vi "Main Page.vi"(8 "error in (no error)":errorcluster, 11 "Node Ptr":T2 format="%.0x") -> (0 "error out":errorcluster)   [LabVIEW 2014, in "SLSC configuration System Explorer.lvlib"]
uses:
  SLSC configuration System Explorer.lvlib
  <vilib>/NI Veristand/Custom Device API/Custom Device Item Ref.ctl
  Shared/Type Defs/RIO Device Address.ctl
  Type Defs/Card Position.ctl
  Example/SPI Utility/Slot #.ctl
  <vilib>/NI Veristand/Custom Device API/Dependent File Optional Info.ctl
  Shared/Constants.vi
  <vilib>/NI Veristand/Custom Device API/Get Item Property (U16).vi
  <vilib>/NI Veristand/Custom Device API/Get Item Property (U32).vi
  <vilib>/NI Veristand/Custom Device API/Get Item Property (Dependent File).vi
  <vilib>/NI Veristand/Custom Device API/Get Item Property (String).vi
  <vilib>/NI Veristand/Custom Device API/Set Item Property (U16).vi
  <vilib>/NI Veristand/Custom Device API/Set Item Property (U32).vi
  <vilib>/NI Veristand/Custom Device API/Set Item Property (Dependent File).vi
  <vilib>/NI Veristand/Custom Device API/Set Item Property (String).vi
  <vilib>/NI Veristand/Custom Device API/Custom Device API.lvlib
  Shared/SLSC configuration Shared.lvlib
panel:
  in  "Header 5":cluster{"Section Name":string}={"Section Name"="Slot Configuration"}
  out "Slot Configuration":string[][](table)
  out "SPI Clock Frequency (Hz)":dbl
  in  "Sample Rate (S/s)":u32 min=1 max=40000000
  in  "FPGA Load Delay (s)":u8
  in  "SPI Divide Value":u8 min=1
  in  "Header 4":cluster{"Section Name":string}={"Section Name"="SPI Configuration"}
  in  "Header 3":cluster{"Section Name":string}={"Section Name"="FPGA Configuration"}
  in  "Header 2":cluster{"Section Name":string}={"Section Name"="Device Settings"}
  in  "RIO Device Address":T1="RIO0"
  in  "Path":path
  in  "Header":cluster{"Section Name":string}={"Section Name"="SLSC Custom Device Settings"}
  in  "Name":string
  # "120 MHz"
  # "______________________"
  # "SPI Clock Frequency ="
  # "(Divide Value + 1) x 2"
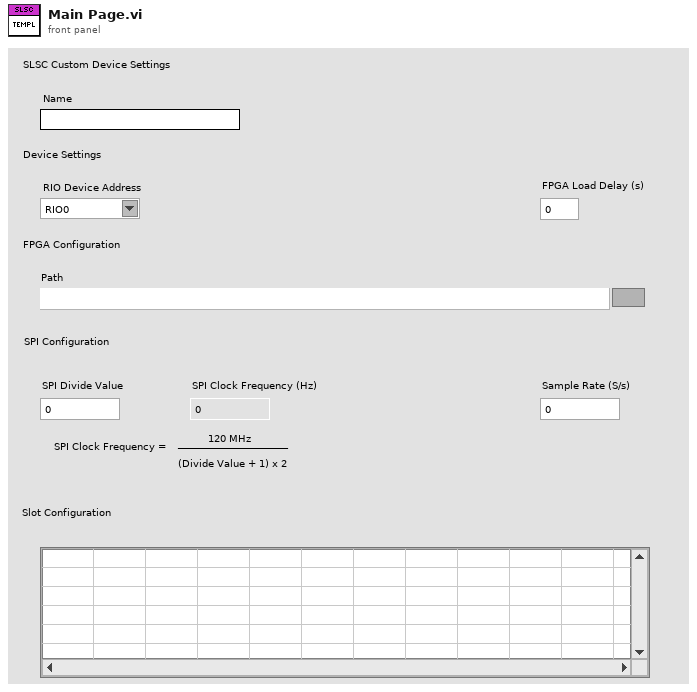
[diagram p1: front panel]
types:
  T1 = typedef "SLSC configuration System Explorer.lvlib/RIO Device Address.ctl" = string
  T2 = typedef "Custom Device API.lvlib/Custom Device Item Ref.ctl" = u64
  T3 = typedef "SLSC configuration Shared.lvlib/Card Position.ctl" = cluster{"Rack #":u8, "Slot #":T4}
  T4 = typedef "SLSC configuration Shared.lvlib/Slot #.ctl" = u8
  T5 = typedef "Custom Device API.lvlib/Custom Device Item Info.ctl" = cluster{"Name":string, "Is Channel":bool, "GUID":string, "Is Waveform":bool}
  T6 = typedef "Custom Device API.lvlib/Dependent File Optional Info.ctl" = cluster{"Version":string, "RTDestination":path, "ForceDownload":bool, "SupportedTarget":string, "MD5":string}
  T7 = typedef "Custom Device API.lvlib/Custom Device Commands.ctl" = enum16{"Default", "Item renamed", "Shutdown", "Dynamic button pressed"}
  T8 = typedef "LVPoint32TypeDef.ctl" = cluster{"Horizontal":i32, "Vertical":i32}
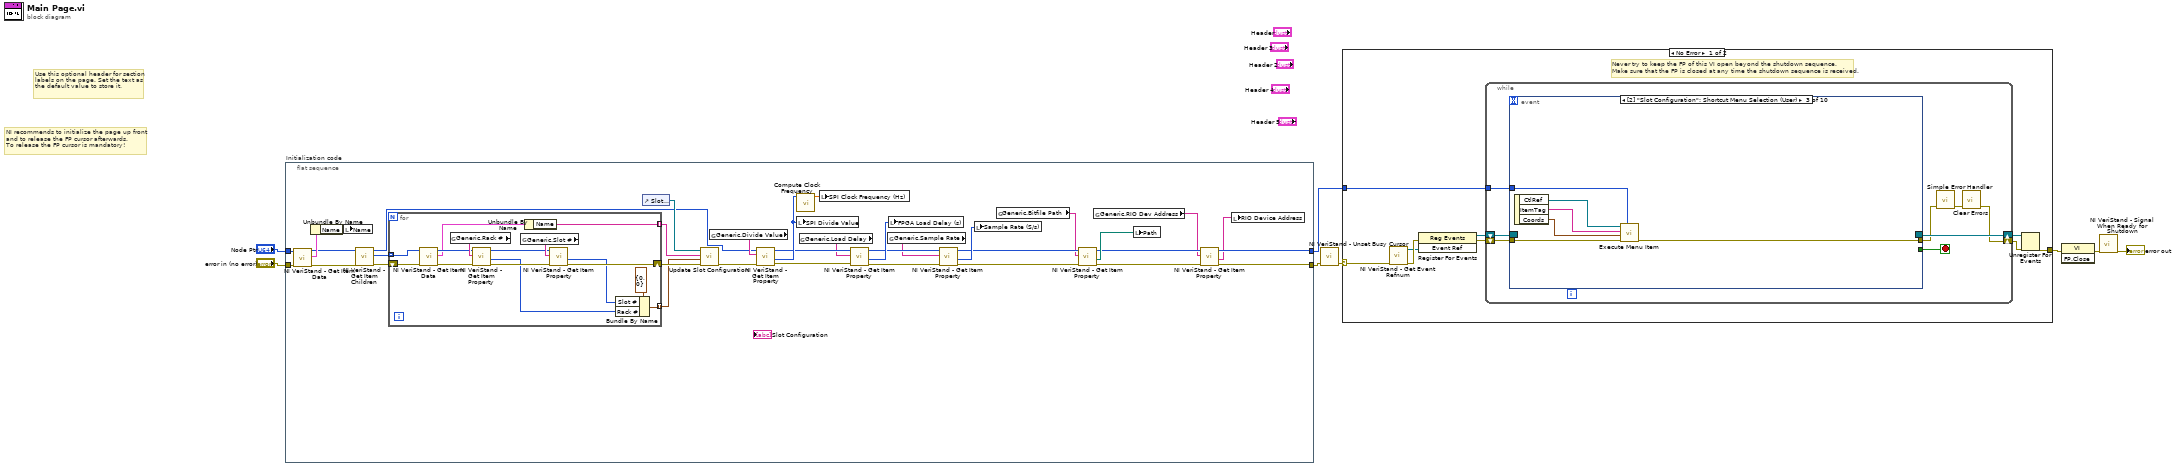
[diagram p0: block diagram]
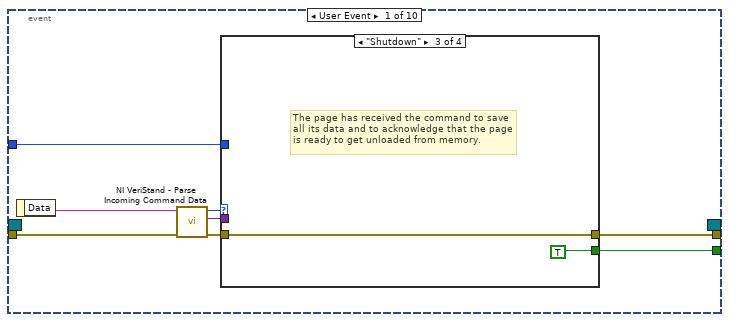
[diagram p2: hidden frame]
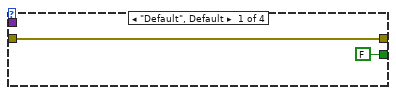
[diagram p3: hidden frame]
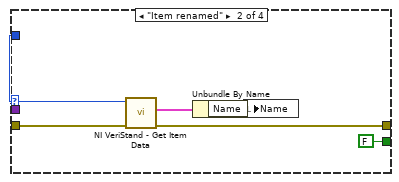
[diagram p4: hidden frame]
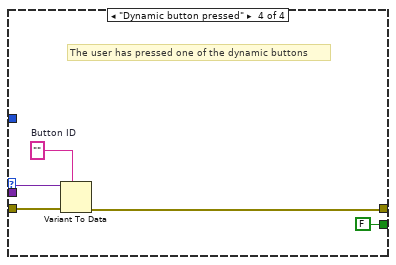
[diagram p5: hidden frame]
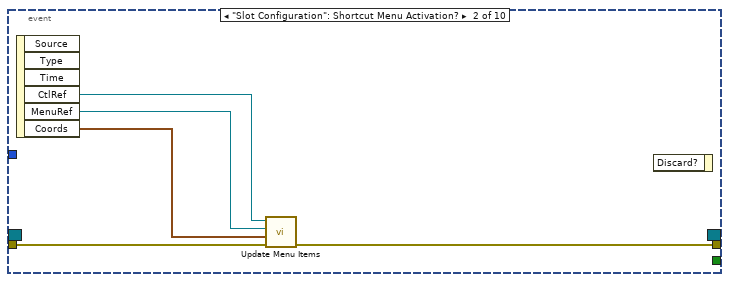
[diagram p6: hidden frame]
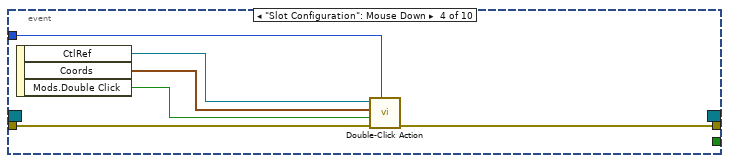
[diagram p7: hidden frame]
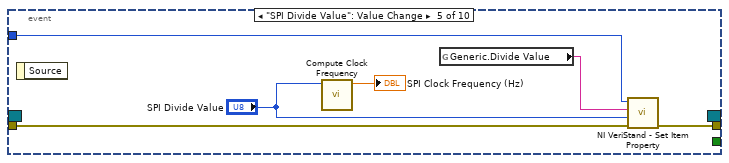
[diagram p8: hidden frame]
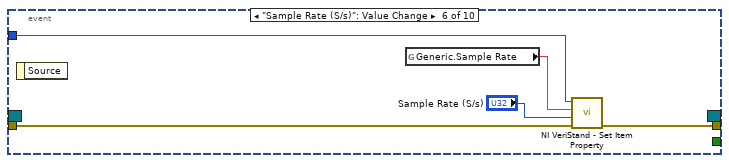
[diagram p9: hidden frame]
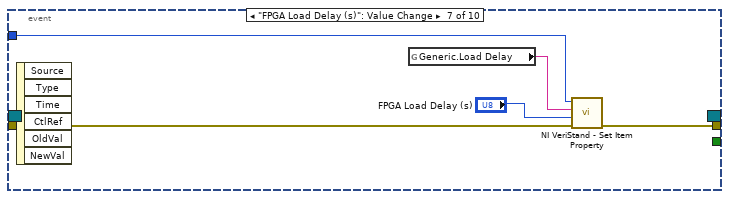
[diagram p10: hidden frame]
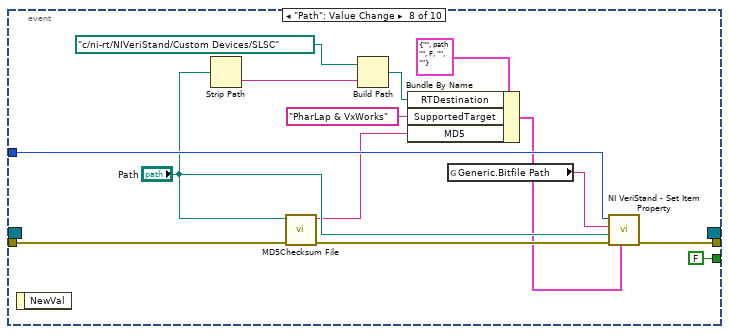
[diagram p11: hidden frame]
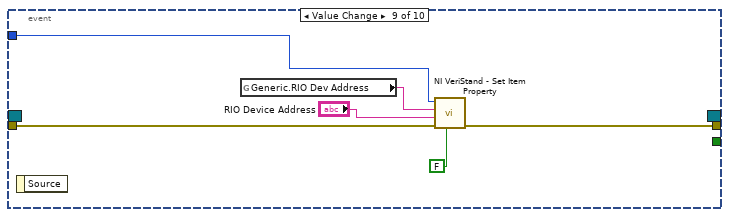
[diagram p12: hidden frame]
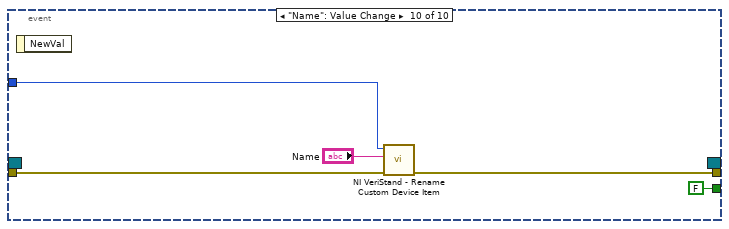
[diagram p13: hidden frame]
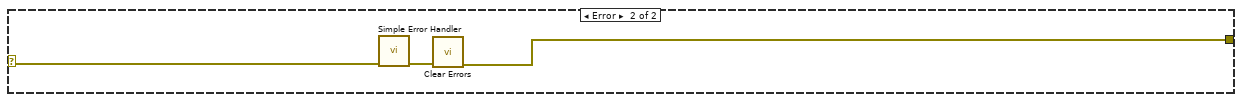
[diagram p14: hidden frame]
diagram:
  # "Use this optional header for section labels on the page. Set the text as the default value to store it."
  # "NI recommends to initialize the page up front\nand to release the FP cursor afterwards.\nTo release the FP cursor is mandatory!"
  n1 = flat-sequence "Initialization code" {
    tunnel: "error in (no error)" -> [w19]
    tunnel: "Node Ptr" -> [w20]
    tunnel: [w23] -> w4
    tunnel: [w22] -> w1
    frame #0 {
      n2 = call <vilib>:"NI VeriStand - Get Item Data.vi"("error in (no error)"=w19, "Item Ref in"=w20) -> ("error out"=w18:errorcluster, "Item Info"=w43:T5, "Item Ref out"=w17:T2)  [unwired: 7 out]
      n3 = Unbundle By Name(w43) -> ("Name"=w42:string)
      n4 = local write "Name"(w42) -> ()
      n5 = call <vilib>:"NI VeriStand - Get Item Children.vi"("error in (no error)"=w18, "Item Ref in"=w17) -> ("error out"=w15:errorcluster, "Child Refs"=w16:T2[], "Item Ref out"=w9:T2)  [unwired: 6 in, 1 out]
      n6 = for {
        tunnel: w16 -> [w53] mode=indexing
        shift-right: [w54] -> w14
        shift-left: w15 -> [w52]
        tunnel: [w48] -> w12 mode=indexing
        tunnel: [w45] -> w11 mode=indexing
        n7 = call <vilib>:"NI VeriStand - Get Item Data.vi"("error in (no error)"=w52, "Item Ref in"=w53) -> ("error out"=w51:errorcluster, "Item Info"=w49:T5, "Item Ref out"=w50:T2)  [unwired: 7 out]
        n8 = global read "Constants.vi" "Generic.Rack #"() -> (w58:string)
        n9 = call-poly <vilib>:"NI VeriStand - Get Item Property.vi"("error in (no error)"=w51, "Property Name"=w58, "Item Ref in"=w50) -> ("error out"=w56:errorcluster, "Value"=w44:u16, "Item Ref out"=w55:T2)  [unwired: 5 in, 1 out]
        n10 = global read "Constants.vi" "Generic.Slot #"() -> (w57:string)
        n11 = Unbundle By Name(w49) -> ("Name"=w48:string)
        n12 = call-poly <vilib>:"NI VeriStand - Get Item Property.vi"("error in (no error)"=w56, "Property Name"=w57, "Item Ref in"=w55) -> ("error out"=w54:errorcluster, "Value"=w46:u16)  [unwired: 5 in, 2 out]
        n13 = Bundle By Name(cluster=T3 {"Rack #"=0, "Slot #"=0} ("Card Position"), "Slot #"=w46, "Rack #"=w44) -> (w45:T3)
      }
      n14 = control-ref of="Slot Configuration"() -> (w13:refnum<vi>)
      n15 = call "Update Slot Configuration.vi"("error in (no error)"=w14, "Card Position"=w11, "Card Name"=w12, "Slot Configuration in"=w13) -> ("error out"=w10:errorcluster)  [unwired: 6 in, 1 out]
      n16 = global read "Constants.vi" "Generic.Divide Value"() -> (w41:string)
      n17 = call-poly <vilib>:"NI VeriStand - Get Item Property.vi"("error in (no error)"=w10, "Property Name"=w41, "Item Ref in"=w9) -> ("error out"=w38:errorcluster, "Value"=w40:u16, "Item Ref out"=w37:T2)  [unwired: 5 in, 1 out]
      n18 = call "Compute Clock Frequency.vi"("SPI Divide Value"=w40) -> ("SPI Clock Frequency (Hz)"=w39:dbl)  [unwired: 10 in]
      n19 = local write "SPI Divide Value"(w40) -> ()
      n20 = global read "Constants.vi" "Generic.Load Delay"() -> (w36:string)
      n21 = local write "SPI Clock Frequency (Hz)"(w39) -> ()
      n22 = call-poly <vilib>:"NI VeriStand - Get Item Property.vi"("error in (no error)"=w38, "Property Name"=w36, "Item Ref in"=w37) -> ("error out"=w34:errorcluster, "Value"=w35:u16, "Item Ref out"=w33:T2)  [unwired: 5 in, 1 out]
      n23 = global read "Constants.vi" "Generic.Sample Rate"() -> (w32:string)
      n24 = local write "FPGA Load Delay (s)"(w35) -> ()
      n25 = call-poly <vilib>:"NI VeriStand - Get Item Property.vi"("error in (no error)"=w34, "Property Name"=w32, "Item Ref in"=w33) -> ("error out"=w30:errorcluster, "Value"=w31:u32, "Item Ref out"=w29:T2)  [unwired: 5 in, 1 out]
      n26 = local write "Sample Rate (S/s)"(w31) -> ()
      n27 = global read "Constants.vi" "Generic.Bitfile Path"() -> (w27:string)
      n28 = call-poly <vilib>:"NI VeriStand - Get Item Property.vi"("error in (no error)"=w30, "Property Name"=w27, "Item Ref in"=w29) -> ("error out"=w26:errorcluster, "Path"=w28:path, "Item Ref out"=w25:T2)  [unwired: 4 in, 2 out]
      n29 = global read "Constants.vi" "Generic.RIO Dev Address"() -> (w24:string)
      n30 = local write "Path"(w28) -> ()
      n31 = call-poly <vilib>:"NI VeriStand - Get Item Property.vi"("error in (no error)"=w26, "Property Name"=w24, "Item Ref in"=w25) -> ("error out"=w23:errorcluster, "Value"=w21:string, "Item Ref out"=w22:T2)  [unwired: 5 in, 1 out]
      n32 = local write "RIO Device Address"(w21) -> ()
    }
  }
  n33 = call <vilib>:"NI VeriStand - Unset Busy Cursor.vi"("error in (no error)"=w4) -> ("error out"=w3:errorcluster)  [unwired: 10 out]
  n34 = case shown="No Error" w3 {
    selector: w3 -> [w59 w159]
    tunnel: [w64 w157] -> w8
    tunnel: w1 -> [w60 _]
    frame No Error {
      # "Never try to keep the FP of this VI open beyond the shutdown sequence.\nMake sure that the FP is closed at any time the shutdown sequence is received."
      n35 = call <vilib>:"NI VeriStand - Get Event Refnum.vi"("error in (no error)"=w59) -> ("error out"=w67:errorcluster, "Event Ref"=w63:refnum<user-event>)  [unwired: 9 out]
      n36 = register-events(error in=w67, w63) -> (reference out=w61:refnum<event-registration>, error out=w62:errorcluster)  [unwired: 1 in]
      n37 = while {
        tunnel: w60 -> [w71]
        shift-right: [w68] -> w65
        shift-left: w62 -> [w74]
        shift-right: [w75] -> w66
        shift-left: w61 -> [w73]
        stop <- w72 stop-if-true
        n38 = event shown="[2] \"Slot Configuration\": Shortcut Menu Selection (User)" {
          selector: w73 -> [_ _ _ _ _ _ _ _ _ _]
          dyn-events: [_ _ _ _ _ _ _ _ _ _] -> w75
          timeout: _ -> [_ _ _ _ _ _ _ _ _ _]
          tunnel: w74 -> [w83 w101 w109 w115 w119 w126 w131 w135 w150 w156]
          tunnel: [w79 _ _ _ _ _ _ FALSE _ FALSE] -> w72
          tunnel: [w78 w100 w104 w110 w118 w125 w130 w143 w149 w155] -> w70
          tunnel: w71 -> [w77 _ w105 w111 w120 w124 w129 w145 w148 w154]
          event User Event {
            n39 = event-data() -> ("Data"=w82:string)  [unwired: 1 out]
            n40 = call <vilib>:"NI VeriStand - Parse Incoming Command Data.vi"("error in (no error)"=w83, "Incoming data"=w82) -> ("error out"=w81:errorcluster, "Outgoing data"=w76:variant, "Action"=w80:T7)  [unwired: 7 out]
            n41 = case shown="\"Shutdown\"" w80 {
              tunnel: w81 -> [w85 w91 w92 w98]
              tunnel: [FALSE FALSE TRUE FALSE] -> w79
              tunnel: [w85 w88 w92 w95] -> w78
              tunnel: w77 -> [_ w90 _ _]
              tunnel: w76 -> [_ _ _ w97]
              frame "Default", Default {
              }
              frame "Item renamed" {
                n42 = call <vilib>:"NI VeriStand - Get Item Data.vi"("error in (no error)"=w91, "Item Ref in"=w90) -> ("error out"=w88:errorcluster, "Item Info"=w89:T5)  [unwired: 8 out]
                n43 = Unbundle By Name(w89) -> ("Name"=w87:string)
                n44 = local write "Name"(w87) -> ()
              }
              frame "Shutdown" {
                # "The page has received the command to save all its data and to acknowledge that the page is ready to get unloaded from memory."
              }
              frame "Dynamic button pressed" {
                w96 = ""  # Button ID
                # "The user has pressed one of the dynamic buttons"
                n45 = Variant To Data(error in=w98, type=w96, Variant=w97) -> (error out=w95:errorcluster)  [unwired: 1 out]
              }
            }
          }
          event "Slot Configuration": Shortcut Menu Activation? {
            n46 = event-data() -> ("CtlRef"=w103:refnum<vi>, "MenuRef"=w99:refnum<k9>, "Coords"=w102:T8)  [unwired: 4 out]
            n47 = call "Update Menu Items.vi"("error in (no error)"=w101, "Coords"=w102, "MenuRef"=w99, "Table in"=w103) -> ("error out"=w100:errorcluster)  [unwired: 7 in]
            n48 = event-data() -> ()  [unwired: 2 in, 1 out]
          }
          event "Slot Configuration": Shortcut Menu Selection (User) {
            n49 = event-data() -> ("CtlRef"=w106:refnum<vi>, "ItemTag"=w107:string, "Coords"=w108:T8)  [unwired: 1 out]
            n50 = call "Execute Menu Item.vi"("Device Ref in"=w105, "error in (no error)"=w109, "Coords"=w108, "ItemTag"=w107, "CtlRef"=w106) -> ("error out"=w104:errorcluster)  [unwired: 6 in]
          }
          event "Slot Configuration": Mouse Down {
            n51 = event-data() -> ("CtlRef"=w112:refnum<vi>, "Coords"=w113:T8, "Mods.Double Click"=w114:bool)  [unwired: 1 out]
            n52 = call "Double-Click Action.vi"("Device Ref in"=w111, "error in (no error)"=w115, "Mods.Double Click"=w114, "Coords"=w113, "CtlRef"=w112) -> ("error out"=w110:errorcluster)  [unwired: 6 in]
          }
          event "SPI Divide Value": Value Change {
            n53 = event-data() -> ()  [unwired: 2 out]
            n54 = call "Compute Clock Frequency.vi"("SPI Divide Value"="SPI Divide Value") -> ("SPI Clock Frequency (Hz)"=→"SPI Clock Frequency (Hz)":dbl)  [unwired: 10 in]
            n55 = global read "Constants.vi" "Generic.Divide Value"() -> (w121:string)
            n56 = call-poly <vilib>:"NI VeriStand - Set Item Property.vi"("error in (no error)"=w119, "Value"="SPI Divide Value", "Property Name"=w121, "Item Ref in"=w120) -> ("error out"=w118:errorcluster)  [unwired: 5 in, 2 out]
          }
          event "Sample Rate (S/s)": Value Change {
            n57 = event-data() -> ()  [unwired: 2 out]
            n58 = global read "Constants.vi" "Generic.Sample Rate"() -> (w123:string)
            n59 = call-poly <vilib>:"NI VeriStand - Set Item Property.vi"("error in (no error)"=w126, "Value"="Sample Rate (S/s)", "Property Name"=w123, "Item Ref in"=w124) -> ("error out"=w125:errorcluster)  [unwired: 5 in, 2 out]
          }
          event "FPGA Load Delay (s)": Value Change {
            n60 = event-data() -> ()  [unwired: 7 out]
            n61 = global read "Constants.vi" "Generic.Load Delay"() -> (w128:string)
            n62 = call-poly <vilib>:"NI VeriStand - Set Item Property.vi"("error in (no error)"=w131, "Value"="FPGA Load Delay (s)", "Property Name"=w128, "Item Ref in"=w129) -> ("error out"=w130:errorcluster)  [unwired: 5 in, 2 out]
          }
          event "Path": Value Change {
            n63 = event-data() -> ()  [unwired: 2 out]
            n64 = Strip Path(path="Path") -> (name=w139:string)  [unwired: 1 out]
            n65 = call <vilib>:"MD5Checksum File.vi"("error in (no error)"=w135, "Path"="Path") -> ("error out"=w134:errorcluster, "MD5 message-digest"=w133:string)  [unwired: 8 in]
            n66 = Build Path(base path=path "c:/ni-rt/NIVeriStand/Custom Devices/SLSC", name or relative path=w139) -> (appended path=w137:path)
            n67 = Bundle By Name(cluster=T6 {"Version"="", "RTDestination"=path "", "ForceDownload"=FALSE, "SupportedTarget"="", "MD5"=""} ("OptionalInfo"), "RTDestination"=w137, "SupportedTarget"="PharLap & VxWorks", "MD5"=w133) -> (w132:T6)
            n68 = global read "Constants.vi" "Generic.Bitfile Path"() -> (w144:string)
            n69 = call-poly <vilib>:"NI VeriStand - Set Item Property.vi"("OptionalInfo"=w132, "error in (no error)"=w134, "Path"="Path", "Property Name"=w144, "Item Ref in"=w145) -> ("error out"=w143:errorcluster)  [unwired: 4 in, 2 out]
          }
          event Value Change {
            n70 = event-data() -> ()  [unwired: 2 out]
            n71 = global read "Constants.vi" "Generic.RIO Dev Address"() -> (w151:string)
            n72 = call-poly <vilib>:"NI VeriStand - Set Item Property.vi"("Binary String (T)"=FALSE, "error in (no error)"=w150, "Value"="RIO Device Address", "Property Name"=w151, "Item Ref in"=w148) -> ("error out"=w149:errorcluster)  [unwired: 4 in, 2 out]
          }
          event "Name": Value Change {
            n73 = event-data() -> ()  [unwired: 2 out]
            n74 = call <vilib>:"NI VeriStand - Rename Custom Device Item.vi"("error in (no error)"=w156, "New Name"="Name", "Item Ref in"=w154) -> ("error out"=w155:errorcluster)  [unwired: 1 in, 7 out]
          }
        }
        n75 = call <vilib>:"Simple Error Handler.vi"("error in (no error)"=w70) -> ("error out"=w69:errorcluster)  [unwired: 1 in, 7 out]
        n76 = call <vilib>:"Clear Errors.vi"("error in (no error)"=w69) -> ("error out"=w68:errorcluster)  [unwired: 1 in, 5 out]
      }
      n77 = Unregister For Events(event registration refnum=w66, error in=w65) -> (error out=w64:errorcluster)
    }
    frame Error {
      n78 = call <vilib>:"Simple Error Handler.vi"("error in (no error)"=w159) -> ("error out"=w158:errorcluster)  [unwired: 1 in, 7 out]
      n79 = call <vilib>:"Clear Errors.vi"("error in (no error)"=w158) -> ("error out"=w157:errorcluster)  [unwired: 1 in, 5 out]
    }
  }
  n80 = invoke class="VI" method="FP.Close"(error in=w8) -> (error out=w7:errorcluster)  [unwired: 2 in, 2 out]
  n81 = call <vilib>:"NI VeriStand - Signal When Ready for Shutdown.vi"("error in (no error)"=w7) -> ("error out"=→"error out":errorcluster)  [unwired: 10 out]
